vi "Set Function B.vi"(9 "function B (deg q:0)":i16(slide) scale=0.0..2.0 scale format="%.2f", 11 "GPIB addess":string="17") -> ()   [LabVIEW 2009, in "HP4192A IA.lvclass"]
uses:
  HP4192A IA.lvclass
panel:
  # "Z/Y   L&C"
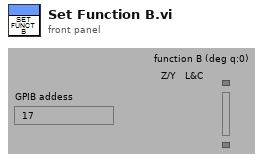
[diagram p1: front panel]
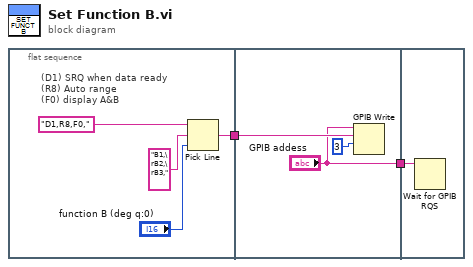
[diagram p0: block diagram]
diagram:
  n1 = flat-sequence {
    tunnel: [w5] -> w2
    tunnel: w2 -> [w8]
    tunnel: ["GPIB addess"] -> w1
    tunnel: w1 -> [w10]
    frame #0 {
      # "(D1) SRQ when data ready\n(R8) Auto range\n(F0) display A&B"
      n2 = Pick Line(string ("")="D1,R8,F0,", multi-line string="B1,\rB2,\rB3,", line index="function B (deg q:0)") -> (output string=w5:string)
    }
    frame #1 {
      n3 = GPIB Write(0:"GPIB addess", 1:w8, 2:3) -> ()  [unwired: 2 in, 2 out]
    }
    frame #2 {
      n4 = Wait for GPIB RQS(4:w10) -> ()  [unwired: 2 in, 2 out]
    }
  }
